vi "RH_FGEN_CreateMultiSine_CustomPhase.vi"(8 "error in (no error)":errorcluster, 10 "Phase 0":bool, 11 "FGEN Parameters":T1 {"Trigger Mode" items=["Single", "Continuous", "Stepped", "Burst"]}) -> (0 "error out":errorcluster, 3 "sine wave":dbl[](array[numeric]))   [LabVIEW 2023, in "ResourceHandling.lvlib"]
doc: "Generates Multi Sine samples"
uses:
  ResourceHandling.lvlib
  TypeDefs/RH_FGEN_Parameters.ctl
  <instrlib>/niFgen/niFgen.llb/niFgen Trigger Mode.ctl
  <vilib>/Analysis/1siggen.llb/Ramp Pattern by Delta.vi
  <vilib>/Analysis/NI_AALBase.lvlib
  <vilib>/measure/NI_MAPro.lvlib
panel:
  out "Waveform Graph":waveform(dbl)(graph)
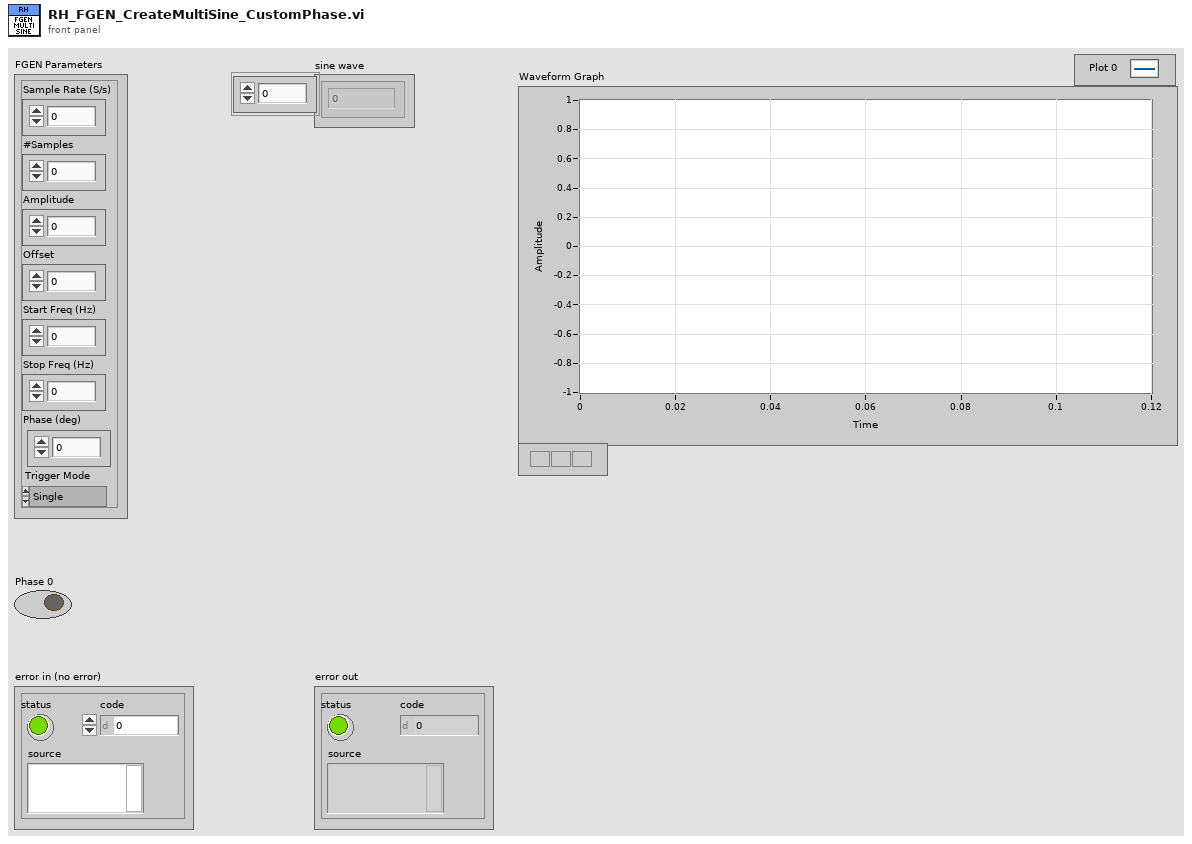
[diagram p1: front panel]
types:
  T1 = typedef "ResourceHandling.lvlib/RH_FGEN_Parameters.ctl" = cluster{"Sample Rate (S/s)":dbl, "#Samples":i32, "Amplitude":dbl, "Offset":dbl, "Start Freq (Hz)":dbl, "Stop Freq (Hz)":dbl, "Phase (deg)":dbl, "Trigger Mode":T2}
  T2 = typedef "niFgen Trigger Mode.ctl" = i32
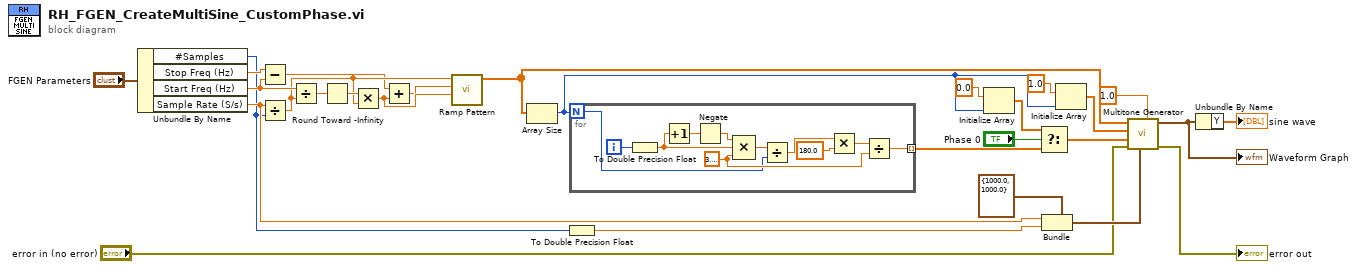
[diagram p0: block diagram]
diagram:
  n1 = Unbundle By Name("FGEN Parameters") -> ("#Samples"=w13:i32, "Stop Freq (Hz)"=w28:dbl, "Start Freq (Hz)"=w27:dbl, "Sample Rate (S/s)"=w14:dbl)
  n2 = Subtract(x=w28, y=w27) -> (x-y=w22:dbl)
  n3 = Divide(x=w14, y=w13) -> (x/y=w24:dbl)
  n4 = Divide(x=w27, y=w24) -> (x/y=w26:dbl)
  n5 = Round Toward -Infinity(1:w26) -> (0:w25:dbl)
  n6 = Multiply(x=w25, y=w24) -> (x*y=w23:dbl)
  n7 = Add(x=w22, y=w23) -> (x+y=w21:dbl)
  n8 = call-poly <vilib>:"Ramp Pattern.vi"("start"=w23, "end"=w21, "delta"=w24) -> ("Ramp Pattern"=w16:dbl[])  [unwired: 6 in, 2 out]
  n9 = Array Size(array=w16) -> (size(s)=w11:i32)
  n10 = To Double Precision Float(number=w13) -> (double precision float=w10:dbl)
  n11 = for {
    N: w11 -> [w30]
    tunnel: [w33] -> w9 mode=indexing
    i -> [w39]
    w31 = 3.141592653589793
    n12 = To Double Precision Float(number=w39) -> (double precision float=w32:dbl)
    n13 = Increment(x=w32) -> (x+1=w38:dbl)
    n14 = Negate(x=w38) -> (-x=w37:dbl)
    n15 = Compound Arithmetic op=MULTIPLY(w37, w32, w31) -> (w36:dbl)
    n16 = Divide(x=w36, y=w30) -> (x/y=w29:dbl)
    n17 = Multiply(x=w29, y=180.0) -> (x*y=w34:dbl)
    n18 = Divide(x=w34, y=w31) -> (x/y=w33:dbl)
  }
  n19 = Initialize Array(0.0 ("element"), w11) -> (w7:dbl[])
  n20 = Select(t=w7, s="Phase 0", f=w9) -> (s? t:f=w8:dbl[])
  n21 = Bundle(cluster=cluster{"Fs":dbl, "#s":dbl} {"Fs"=1000.0, "#s"=1000.0} ("sampling info"), "Fs"=w14, "#s"=w10) -> (w12:cluster{"Fs":dbl, "#s":dbl})
  n22 = Initialize Array(1.0 ("amplitude"), w11) -> (w18:dbl[])
  n23 = call <vilib>:"Multitone Generator.vi"("amplitude"=1.0, "sampling info"=w12, "error in (no error)"="error in (no error)", "tone phases"=w8, "tone amplitudes"=w18, "tone frequencies"=w16) -> ("error out"=→"error out":errorcluster, "signal out"=w4:waveform(dbl))  [unwired: 2 in, 2 out]
  "Waveform Graph" <- w4
  n24 = Unbundle By Name(w4) -> ("Y"=→"sine wave":dbl[])
